vi "RSZVB Set Connector.vi"(7 "Connector (0: N 50 Ohm (f))":i32(ring) items=["N 50 Ohm (f)", "N 50 Ohm (m)", "N 75 Ohm (f)", "N 75 Ohm (m)", "PC 7", "PC 3.5 (f)", "PC 3.5 (m)", "2.92 mm (f)", "2.92 mm (m)", "2.4 mm (f)", "2.4 mm (m)", "1.85 mm (f)", "1.85 mm (m)", "7-16 (f)", "7-16 (m)", "PC 1 (f)", "PC 1 (m)", "PC 1.85 (f)", "PC 1.85 (m)", "PC 2.4 (f)", "PC 2.4 (m)"], 8 "error in (no error)":errorcluster {"code" format="%.0x"}, 9 "Port (1)":i32=1, 10 "Channel (1)":i32=1, 11 "VISA session":refnum<visa-resource-name>) -> (0 "error out":errorcluster {"code" format="%.0x"}, 3 "dup VISA session":refnum<visa-resource-name>)   [LabVIEW 2011]
doc: "This VI selects a connector type at a specified port <Port> and its gender.\n\nRemote-control command(s):\n[SENSe<Ch>:]CORRection:COLLect:CONNection<port_no> N50FEMALE | N50MALE | N75FEMALE | N75MALE | PC7 | PC35FEMALE | PC35MALE | PC292FEMALE | PC292MALE | UFEMALE1 | UMALE1 | UFEMALE2 | UMALE2 | SMAFEMALE | SMAMALE | PC1FEMALE | PC1MALE | PC185FEMALE | PC185MALE | PC24FEMALE | PC24MALE"
uses:
  _utility/RSZVB Global Data.vi
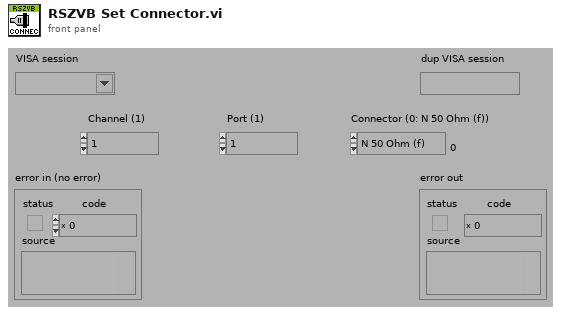
[diagram p1: front panel]
types:
  T1 = cluster{"Error Checking (T: On)":bool, "Installed Options":string[], "Data Valid?":bool, "Ports":i32, "Model":string[], "Option Checking (T: On)":bool}[]
  T2 = cluster{"Error Checking (T: On)":bool, "Installed Options":string[], "Data Valid?":bool, "Ports":i32, "Model":string[], "Option Checking (T: On)":bool}
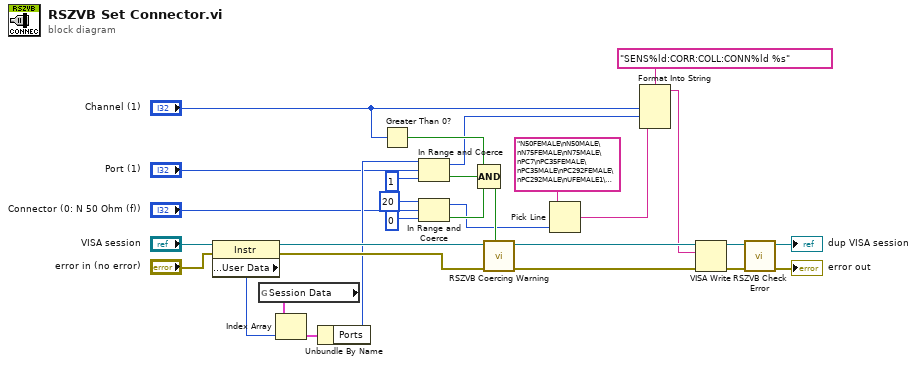
[diagram p0: block diagram]
diagram:
  n1 = property class="Instr"(reference="VISA session", error in="error in (no error)") -> (reference out=w16:refnum<visa-resource-name>, error out=w17:errorcluster, "General Settings:User Data"=w18:u32)
  n2 = global read "RSZVB Global Data.vi" "Session Data"() -> (w19:T1)
  n3 = Index Array(array=w19, index=w18) -> (element=w20:T2)
  n4 = Unbundle By Name(w20) -> ("Ports"=w8:i32)
  n5 = Greater Than 0?(x="Channel (1)") -> (x > 0?=w21:bool)
  n6 = In Range and Coerce(upper limit=w8, x="Port (1)", lower limit=1) -> (coerced(x)=w4:i32, In Range?=w24:bool)
  n7 = In Range and Coerce(upper limit=20 ("lower limit"), x="Connector (0: N 50 Ohm (f))", lower limit=0) -> (coerced(x)=w2:i32, In Range?=w14:bool)
  n8 = Compound Arithmetic op=AND(w21, w24, w14) -> (w23:bool)
  n9 = call "RSZVB Coercing Warning.vi"("In Range?"=w23, "error in (no error)"=w17, "VISA session"=w16) -> ("error out"=w27:errorcluster, "dup VISA session"=w28:refnum<visa-resource-name>)  [unwired: 7 in]
  n10 = Pick Line(multi-line string="N50FEMALE\nN50MALE\nN75FEMALE\nN75MALE\nPC7\nPC35FEMALE\nPC35MALE\nPC292FEMALE\nPC292MALE\nUFEMALE1\nUMALE1\nUFEMALE2\nUMALE2\nSMAFEMALE\nSMAMALE\nPC1FEMALE\nPC1MALE\nPC185FEMALE\nPC185MALE\nPC24FEMALE\nPC24MALE", line index=w2) -> (output string=w1:string)  [unwired: 1 in]
  n11 = Format Into String(format string="SENS%ld:CORR:COLL:CONN%ld %s", "Channel (1)", w4, w1) -> (resulting string=w22:string)  [unwired: 2 in, 1 out]
  n12 = VISA Write(VISA resource name=w28, write buffer=w22, error in (no error)=w27) -> (VISA resource name out=w25:refnum<visa-resource-name>, error out=w26:errorcluster)  [unwired: 1 out]
  n13 = call "RSZVB Check Error.vi"("error in (no error)"=w26, "VISA session"=w25) -> ("error out"=→"error out":errorcluster, "dup VISA session"=→"dup VISA session":refnum<visa-resource-name>)  [unwired: 8 in]
